vi "Seq Dialog Anti Pinch Limits.vi"(8 "Segment Data":T1, 11 "Station":enum16{"Pre Run", "Audit"}(ring)) -> (0 "Step Hisitory":string[](array[string]), 2 "Segment Data 2":T1)   [LabVIEW 2018]
uses:
  type defs/Sequence Info.ctl
  type defs/Anti Pinch Test Data Control.ctl
panel:
  in  "Vent Max Reversal Force":dbl=200.0
  in  "Rollo02 Max Reversal Force":dbl=200.0
  out "error out":errorcluster
  in  "Rollo Max Reversal Force":dbl=200.0
  in  "Glass  Max Reversal Force":dbl=200.0
  out "String 2":string="Pre Run Station - Glass - Vent Open"
  in  "Power Supply Voltage":dbl=10.0
  in  "Description":string
  in  "Save":bool
  in  "Cancel":bool
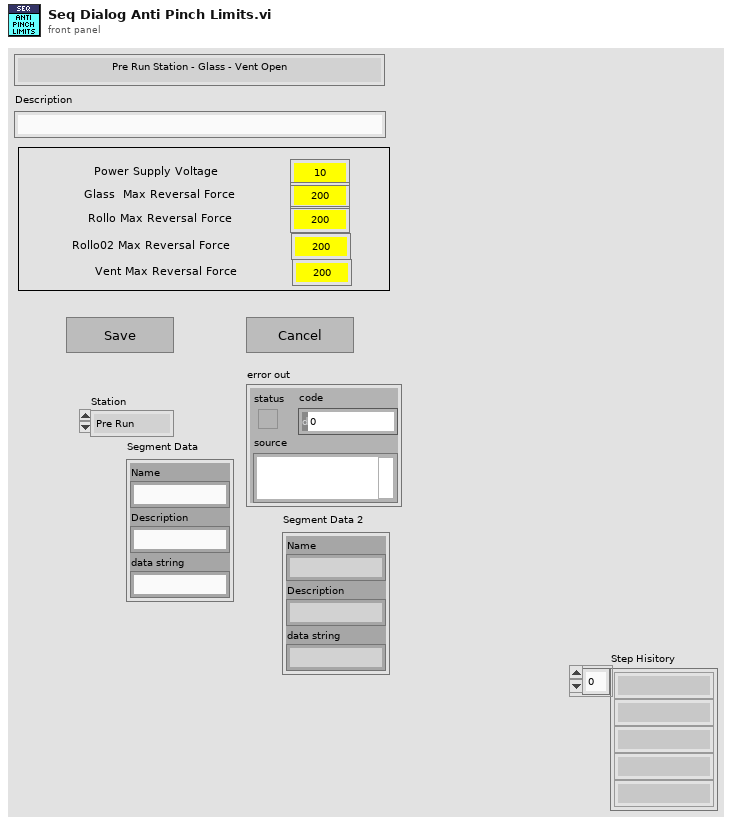
[diagram p1: front panel]
types:
  T1 = typedef "Sequence Info.ctl" = cluster{"Name":string, "Description":string, "data string":string}
  T2 = typedef "Anti Pinch Test Data Control.ctl" = cluster{"Power Supply Voltage":dbl, "Glass  Max Reversal Force":dbl, "Rollo Max Reversal Force":dbl, "Rollo02 Max Reversal Force":dbl, "Vent Max Reversal Force":dbl}
  T3 = cluster{"Anti Pinch Test Data Control":T2, "Segment Data":T1, "Old Data":string, "New Data":string}
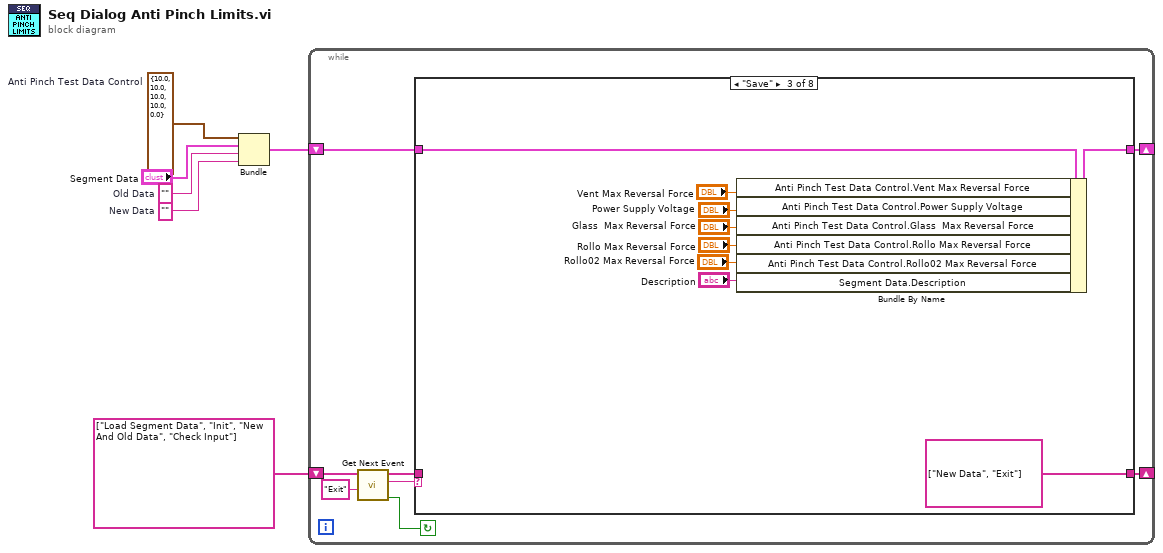
[diagram p0: block diagram]
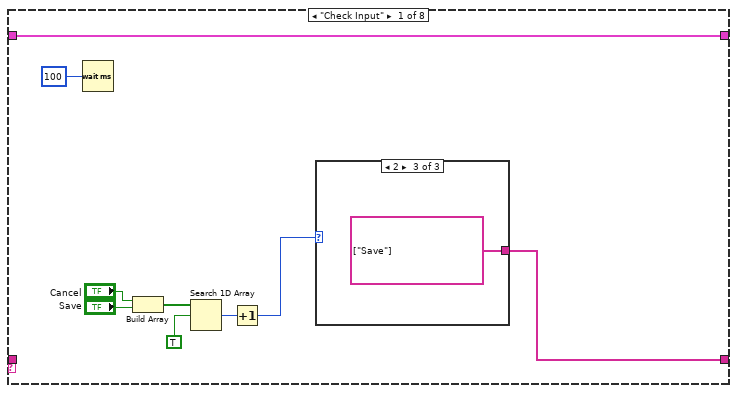
[diagram p2: hidden frame]
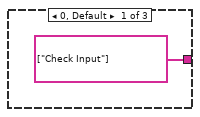
[diagram p3: hidden frame]
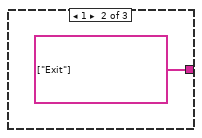
[diagram p4: hidden frame]
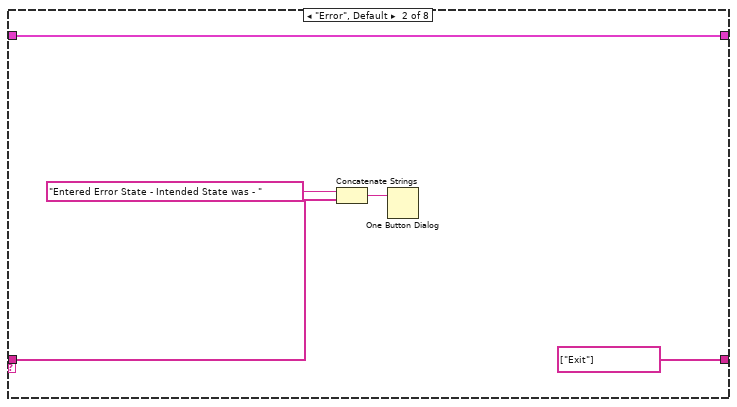
[diagram p5: hidden frame]
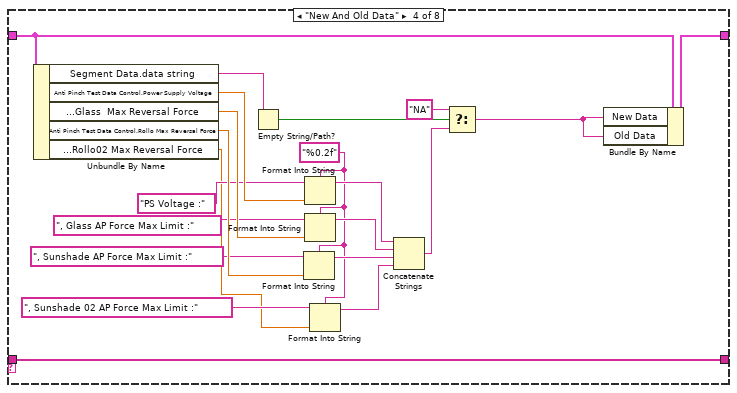
[diagram p6: hidden frame]
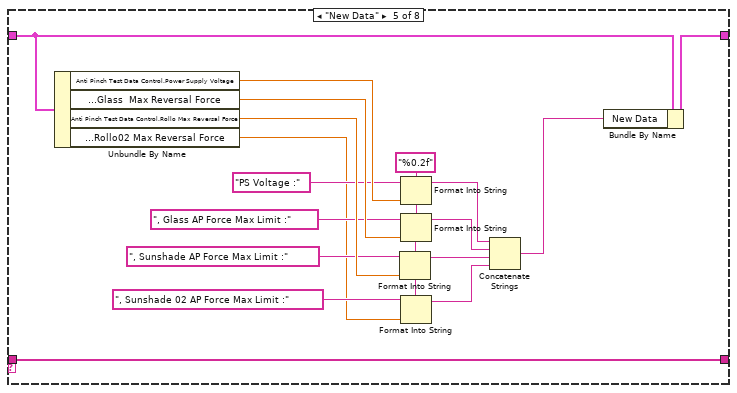
[diagram p7: hidden frame]
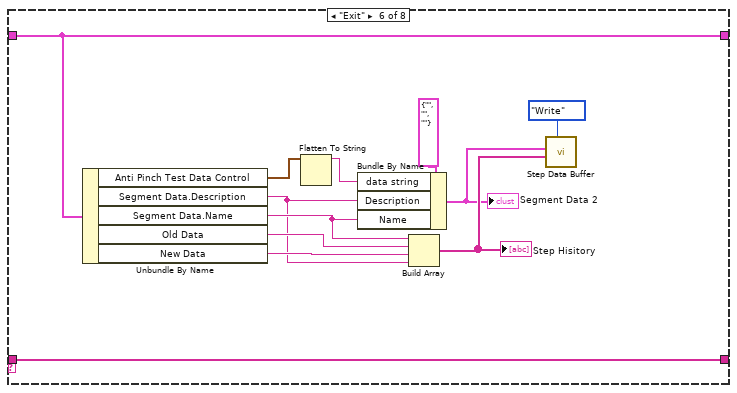
[diagram p8: hidden frame]
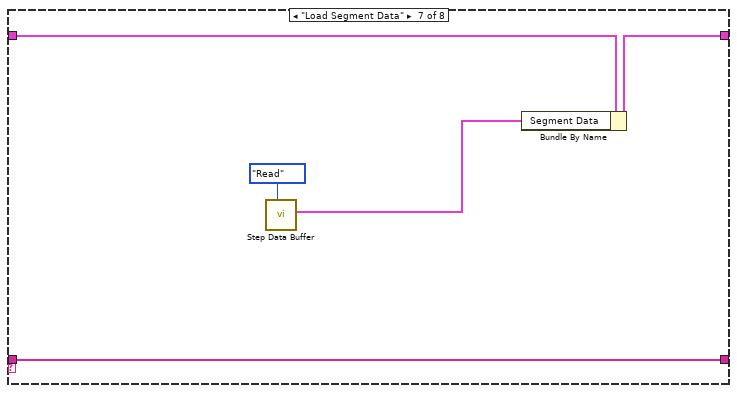
[diagram p9: hidden frame]
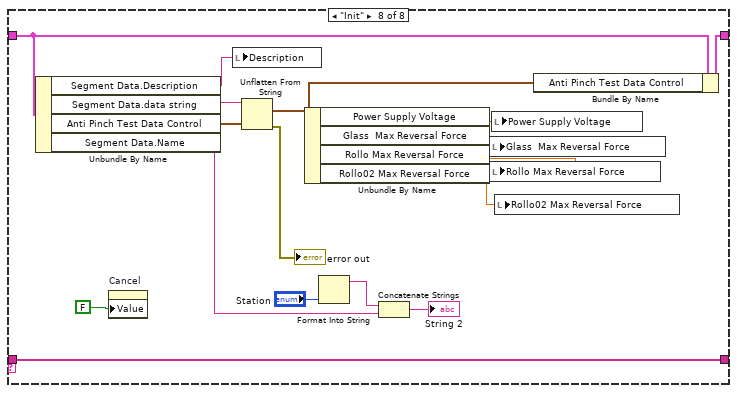
[diagram p10: hidden frame]
diagram:
  w2 = ""  # New Data
  w3 = ""  # Old Data
  w4 = T2 {"Power Supply Voltage"=10.0, "Glass  Max Reversal Force"=10.0, "Rollo Max Reversal Force"=10.0, "Rollo02 Max Reversal Force"=10.0, "Vent Max Reversal Force"=0.0}  # Anti Pinch Test Data Control
  n1 = Bundle("Anti Pinch Test Data Control"=w4, "Segment Data"="Segment Data", "Old Data"=w3, "New Data"=w2) -> (w6:T3)  [unwired: 1 in]
  n2 = while {
    shift-right: [w12] -> _
    shift-left: string[] ["Load Segment Data", "Init", "New And Old Data", "Check Input"] ("Event queue out") -> [w11]
    shift-right: [w7] -> _
    shift-left: w6 -> [w8]
    stop <- w10 continue-if-true
    n3 = call "Get Next Event.vi"("Exit Event"="Exit", "event queue in"=w11) -> ("Condition (Exit:F)"=w10:bool, "next event"=w14:string, "event queue out"=w13:string[])  [unwired: 3 in]
    n4 = case shown="\"Save\"" w14 {
      tunnel: w13 -> [_ w28 _ w49 w71 w89 w95 w109]
      tunnel: [w15 string[] ["Exit"] ("event queue out") string[] ["New Data", "Exit"] ("Event queue out") w49 w71 w89 w95 w109] -> w12
      tunnel: w8 -> [w22 w27 w40 w52 w74 w90 w92 w103]
      tunnel: [w22 w27 w39 w51 w73 w90 w91 w102] -> w7
      frame "Check Input" {
        n5 = Wait (ms)(milliseconds to wait=u32 100) -> ()  [unwired: 1 out]
        n6 = Build Array("Cancel", "Save") -> (w19:bool[])
        n7 = Search 1D Array(1D array=w19, element=TRUE) -> (index of element=w20:i32)  [unwired: 1 in]
        n8 = Increment(x=w20) -> (x+1=w21:i32)
        n9 = case shown="2" w21 {
          tunnel: [string[] ["Check Input"] ("Events to Insert") string[] ["Exit"] ("Events to Insert") string[] ["Save"] ("Events to Insert")] -> w15
          frame 0, Default {
          }
          frame 1 {
          }
          frame 2 {
          }
        }
      }
      frame "Error", Default {
        n10 = Concatenate Strings("Entered Error State - Intended State was - " ("string"), w28) -> (w31:string)
        n11 = One Button Dialog(message=w31) -> ()  [unwired: 1 in, 1 out]
      }
      frame "Save" {
        n12 = Bundle By Name(cluster=w40, "Anti Pinch Test Data Control.Vent Max Reversal Force"="Vent Max Reversal Force", "Anti Pinch Test Data Control.Power Supply Voltage"="Power Supply Voltage", "Anti Pinch Test Data Control.Glass  Max Reversal Force"="Glass  Max Reversal Force", "Anti Pinch Test Data Control.Rollo Max Reversal Force"="Rollo Max Reversal Force", "Anti Pinch Test Data Control.Rollo02 Max Reversal Force"="Rollo02 Max Reversal Force", "Segment Data.Description"="Description") -> (w39:T3)
      }
      frame "New And Old Data" {
        w41 = "%0.2f" ("format string")
        n13 = Unbundle By Name(w52) -> ("Segment Data.data string"=w61:string, "Anti Pinch Test Data Control.Power Supply Voltage"=w56:dbl, "Anti Pinch Test Data Control.Glass  Max Reversal Force"=w54:dbl, "Anti Pinch Test Data Control.Rollo Max Reversal Force"=w50:dbl, "Anti Pinch Test Data Control.Rollo02 Max Reversal Force"=w43:dbl)
        n14 = Empty String/Path?(string/path=w61) -> (empty?=w60:bool)
        n15 = Format Into String(format string=w41, initial string=", Sunshade AP Force Max Limit :" ("string"), w50) -> (resulting string=w48:string)  [unwired: 1 in, 1 out]
        n16 = Format Into String(format string=w41, initial string="PS Voltage :" ("string"), w56) -> (resulting string=w55:string)  [unwired: 1 in, 1 out]
        n17 = Format Into String(format string=w41, initial string=", Glass AP Force Max Limit :" ("string"), w54) -> (resulting string=w53:string)  [unwired: 1 in, 1 out]
        n18 = Format Into String(format string=w41, initial string=", Sunshade 02 AP Force Max Limit :" ("string"), w43) -> (resulting string=w42:string)  [unwired: 1 in, 1 out]
        n19 = Concatenate Strings(w55, w53, w48, w42) -> (w57:string)
        n20 = Select(t="NA", s=w60, f=w57) -> (s? t:f=w58:string)
        n21 = Bundle By Name(cluster=w52, "New Data"=w58, "Old Data"=w58) -> (w51:T3)
      }
      frame "New Data" {
        w65 = "%0.2f" ("format string")
        n22 = Unbundle By Name(w74) -> ("Anti Pinch Test Data Control.Power Supply Voltage"=w78:dbl, "Anti Pinch Test Data Control.Glass  Max Reversal Force"=w76:dbl, "Anti Pinch Test Data Control.Rollo Max Reversal Force"=w72:dbl, "Anti Pinch Test Data Control.Rollo02 Max Reversal Force"=w63:dbl)
        n23 = Format Into String(format string=w65, initial string=", Sunshade AP Force Max Limit :" ("string"), w72) -> (resulting string=w70:string)  [unwired: 1 in, 1 out]
        n24 = Format Into String(format string=w65, initial string="PS Voltage :" ("string"), w78) -> (resulting string=w77:string)  [unwired: 1 in, 1 out]
        n25 = Format Into String(format string=w65, initial string=", Glass AP Force Max Limit :" ("string"), w76) -> (resulting string=w75:string)  [unwired: 1 in, 1 out]
        n26 = Format Into String(format string=w65, initial string=", Sunshade 02 AP Force Max Limit :" ("string"), w63) -> (resulting string=w62:string)  [unwired: 1 in, 1 out]
        n27 = Concatenate Strings(w77, w75, w70, w62) -> (w66:string)
        n28 = Bundle By Name(cluster=w74, "New Data"=w66) -> (w73:T3)
      }
      frame "Exit" {
        n29 = Unbundle By Name(w90) -> ("Anti Pinch Test Data Control"=w88:T2, "Segment Data.Description"=w79:string, "Segment Data.Name"=w83:string, "Old Data"=w85:string, "New Data"=w84:string)
        n30 = Flatten To String(anything=w88) -> (data string=w86:string)  [unwired: 3 in, 2 out]
        n31 = Bundle By Name(cluster=T1 {"Name"="", "Description"="", "data string"=""} ("Segment Data"), "data string"=w86, "Description"=w79, "Name"=w83) -> (w80:T1)
        "Segment Data 2" <- w80
        n32 = Build Array(w83, w85, w84, w79) -> (w81:string[])
        "Step Hisitory" <- w81
        n33 = call "Step Data Buffer.vi"("Mode"=enum16{"Init", "Read", "Write"}."Write", "Step Hisitory In"=w81, "Segment Data In"=w80) -> ()  [unwired: 4 in, 5 out]
      }
      frame "Load Segment Data" {
        n34 = call "Step Data Buffer.vi"("Mode"=enum16{"Init", "Read", "Write"}."Read") -> ("Segment Data Out"=w94:T1)  [unwired: 6 in, 4 out]
        n35 = Bundle By Name(cluster=w92, "Segment Data"=w94) -> (w91:T3)
      }
      frame "Init" {
        n36 = Unbundle By Name(w103) -> ("Segment Data.Description"=w105:string, "Segment Data.data string"=w112:string, "Anti Pinch Test Data Control"=w111:T2, "Segment Data.Name"=w104:string)
        n37 = property on="Cancel" class="Bool (严格)"("Value"=FALSE ("Exit")) -> ()  [unwired: 2 in, 2 out]
        n38 = local write "Description"(w105) -> ()
        n39 = Unflatten From String(type=w111, binary string=w112) -> (value=w101:T2, error out=→"error out":errorcluster)  [unwired: 3 in, 1 out]
        n40 = Unbundle By Name(w101) -> ("Power Supply Voltage"=w110:dbl, "Glass  Max Reversal Force"=w100:dbl, "Rollo Max Reversal Force"=w99:dbl, "Rollo02 Max Reversal Force"=w96:dbl)
        n41 = Format Into String("Station") -> (resulting string=w107:string)  [unwired: 3 in, 1 out]
        n42 = Concatenate Strings(w107, w104) -> (→"String 2":string)
        n43 = local write "Glass  Max Reversal Force"(w100) -> ()
        n44 = local write "Rollo Max Reversal Force"(w99) -> ()
        n45 = local write "Power Supply Voltage"(w110) -> ()
        n46 = local write "Rollo02 Max Reversal Force"(w96) -> ()
        n47 = Bundle By Name(cluster=w103, "Anti Pinch Test Data Control"=w101) -> (w102:T3)
      }
    }
  }
